vi "Update Map with New RT Task Data.vi"(10 "RTOS Data":T1[](array[typedef]) {"CRC" format="%08x"; "Frame Header"."Options" format="%016b"; "Frame Header"."Time" format="%^<%I:%M:%S%3u %p\n%m/%d/%Y %Z>T"; "Frame Header"."Sync" format="%08x"}, 11 "RTOS Map In":map{string, T5[]}(c390)) -> (3 "RTOS Map Out":map{string, T5[]}(c390))   [LabVIEW 2020]
uses:
  Type Definitions/Real Time Task Status.ctl
  Type Definitions/Data Frame.ctl
  Type Definitions/Data Frame Header.ctl
  Type Definitions/Payload Class.ctl
  Type Definitions/Device.ctl
  <vilib>/Utility/miscctls.llb/LVMapReplaceAction.ctl
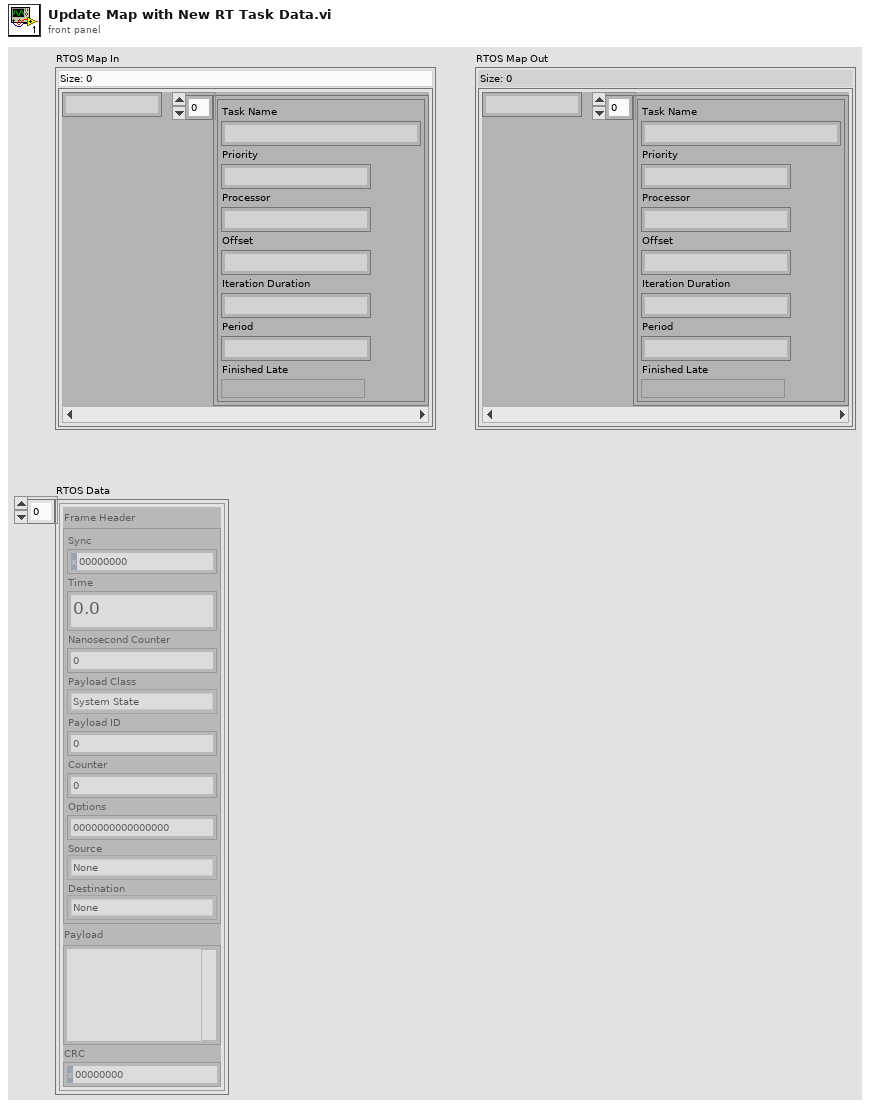
[diagram p1: front panel]
types:
  T1 = typedef "Data Frame.ctl" = cluster{"Frame Header":T2, "Payload":string, "CRC":u32}
  T2 = typedef "Data Frame Header.ctl" = cluster{"Sync":u32, "Time":dbl, "Nanosecond Counter":i64, "Payload Class":T3, "Payload ID":u16, "Counter":i32, "Options":u32, "Source":T4, "Destination":T4}
  T3 = typedef "Payload Class.ctl" = enum16{"System State", "Parameters", "Metadata", "Software Monitor", "Data", "Commands"}
  T4 = typedef "Device.ctl" = enum32{"None", "Exec", "Aux1", "Aux2", "Aux3"}
  T5 = typedef "Real Time Task Status.ctl" = cluster{"Task Name":string, "Priority":i32, "Processor":i32, "Offset":i64, "Iteration Duration":i64, "Period":i64, "Finished Late":bool}
  T6 = typedef "LVMapReplaceAction.ctl" = enum32{"Modify Entry only if found", "Add or Modify Entry", "Delete Entry"}
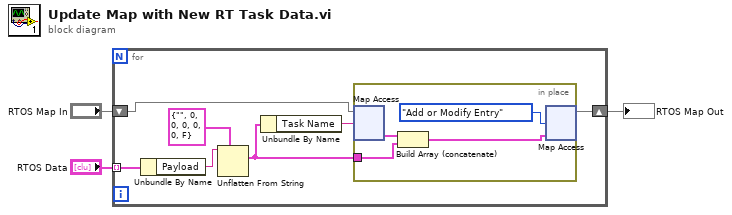
[diagram p0: block diagram]
diagram:
  n1 = for {
    tunnel: "RTOS Data" -> [w10] mode=indexing
    shift-right: [w4] -> w2
    shift-left: "RTOS Map In" -> [w5]
    n2 = Unbundle By Name(w10) -> ("Payload"=w9:string)
    n3 = Unflatten From String(type=T5 {"Task Name"="", "Priority"=0, "Processor"=0, "Offset"=0, "Iteration Duration"=0, "Period"=0, "Finished Late"=FALSE} ("Real Time Task Status"), binary string=w9) -> (value=w6:T5)  [unwired: 3 in, 2 out]
    n4 = Unbundle By Name(w6) -> ("Task Name"=w7:string)
    n5 = in-place {
      in-place-border: w6 -> [w13]
      n6 = in-place-map #1(w5, w7) -> (w14:T5[])  [unwired: 1 in, 1 out]
      n7 = Build Array (concatenate)(w14, w13) -> (w12:T5[])
      n8 = in-place-map #1(w12, LVMapReplaceAction."Add or Modify Entry" ("action")) -> (w4:map{string, T5[]})  [unwired: 2 out]
    }
  }
  "RTOS Map Out" <- w2
